vi "Gyro Change Mode.vi"(8 "error in (no error)":errorcluster, 10 "DPS Mode":T1, 11 "I2CDevRef":T2={"DevStatus"={"status"=FALSE, "code"=0, "source"=""}, "Controller"=enum."Controller 1", "Device Address"=0, "Handle"=0, "I2C Bus"=enum."Invalid"} {"Device Address" format="%.0x"}) -> (0 "error out":errorcluster, 3 "I2CDevRef Out":T2={"DevStatus"={"status"=FALSE, "code"=0, "source"=""}, "Controller"=enum."Controller 1", "Device Address"=0, "Handle"=0, "I2C Bus"=enum."Invalid"} {"Device Address" format="%.0x"})   [LabVIEW 2014]
uses:
  <vilib>/Rock Robotics/WPI/I2C/WPI_I2CDevRef.ctl
  <vilib>/Rock Robotics/SystemInterfaces/Typedef/FPGA_TypedefDigitalModule.ctl
  <vilib>/Rock Robotics/SystemInterfaces/i2clib/i2c_bus.ctl
  DPS Mode.ctl
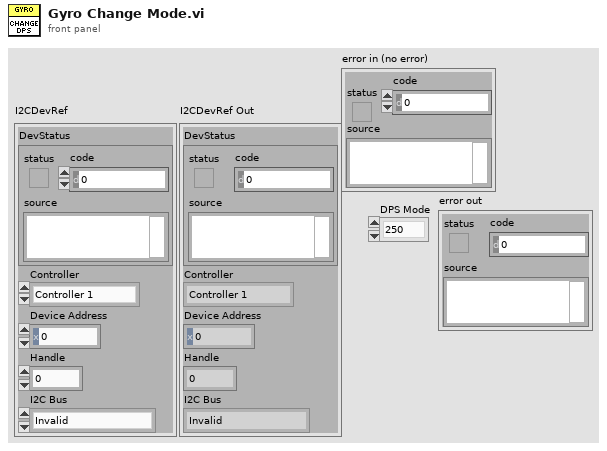
[diagram p1: front panel]
types:
  T1 = typedef "DPS Mode.ctl" = enum16{"250", "500", "2000"}
  T2 = typedef "WPI_I2CDevRef.ctl" = cluster{"DevStatus":errorcluster, "Controller":T3, "Device Address":u8, "Handle":i32, "I2C Bus":T4}
  T3 = typedef "FPGA_TypedefDigitalModule.ctl" = enum16{"Controller 1"}
  T4 = typedef "i2c_bus.ctl" = enum16{"I2C On-Board", "I2C MXP", "Invalid"}
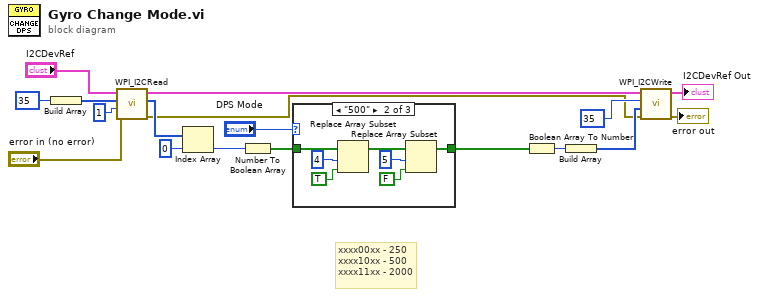
[diagram p0: block diagram]
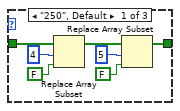
[diagram p2: hidden frame]
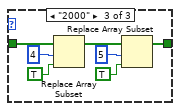
[diagram p3: hidden frame]
diagram:
  # "xxxx00xx - 250\nxxxx10xx - 500\nxxxx11xx - 2000"
  n1 = Build Array(u8 35 ("Data To Send")) -> (w9:u8[])
  n2 = call <vilib>:"WPI_I2CRead.vi"("error in (no error)"="error in (no error)", "I2CBytesToRead"=u8 1, "I2CRegister"=w9, "I2CDevRef"="I2CDevRef") -> ("error out"=w2:errorcluster, "Data Out"=w18:u8[], "I2CDevRef"=w13:T2)  [unwired: 5 in]
  n3 = Index Array(array=w18, index=0) -> (element=w16:u8)
  n4 = Number To Boolean Array(number=w16) -> (Boolean array=w5:bool[])
  n5 = case shown="\"500\"" "DPS Mode" {
    tunnel: w5 -> [w21 w26 w33]
    tunnel: [w19 w27 w34] -> w4
    frame "250", Default {
      n6 = Replace Array Subset(array=w21, new element=FALSE ("new element/subarray"), index=4) -> (w20:bool[])
      n7 = Replace Array Subset(array=w20, new element=FALSE ("new element/subarray"), index=5) -> (w19:bool[])
    }
    frame "500" {
      n8 = Replace Array Subset(array=w26, new element=TRUE ("new element/subarray"), index=4) -> (w28:bool[])
      n9 = Replace Array Subset(array=w28, new element=FALSE ("new element/subarray"), index=5) -> (w27:bool[])
    }
    frame "2000" {
      n10 = Replace Array Subset(array=w33, new element=TRUE ("new element/subarray"), index=4) -> (w35:bool[])
      n11 = Replace Array Subset(array=w35, new element=TRUE ("new element/subarray"), index=5) -> (w34:bool[])
    }
  }
  n12 = Boolean Array To Number(Boolean array=w4) -> (number=w15:u32)
  n13 = Build Array(w15) -> (w14:u32[])
  n14 = call <vilib>:"WPI_I2CWrite.vi"("error in (no error)"=w2, "I2CDataToSend"=w14, "I2CRegister"=u8 35 ("Data To Send"), "I2CDevRef"=w13) -> ("error out"=→"error out":errorcluster, "I2CDevRef"=→"I2CDevRef Out":T2)  [unwired: 6 in]
